vi "MSE310ProjectV2.vi"() -> ()   [LabVIEW 2016]
uses:
  MSE310Project-master/MSE310 Project Control.ctl
  <vilib>/DAQmx/read.llb/DAQmx Read (Digital Bool 1Line 1Point).vi
  <vilib>/DAQmx/write.llb/DAQmx Write (Digital Bool 1Line 1Point).vi
  <vilib>/DAQmx/create/channels.llb/DAQmx Create Channel (DO-Digital Output).vi
  <vilib>/DAQmx/create/channels.llb/DAQmx Create Channel (DI-Digital Input).vi
  <vilib>/DAQmx/miscellaneous.llb/DAQmx Fill In Error Info.vi
panel:
  out "KICK_GT1":bool
  out "HOP_DELAY":u16
  out "TIME_HOP":u16
  out "TIME_CUR":u16
  out "HOPPER-1":bool
  out "HOPPER":bool
  out "HOP_TIME_FLAG":bool
  out "KICK_E1":bool
  out "TOP_PUSH-1":bool
  out "KICK_FLAG-1":bool
  out "KICK_FLAG":bool
  out "KICK_COUNT":u16
  out "HOP_LIT_SENS":bool
  out "TOP_PUSH":bool
  out "RUNNING":bool
  out "START":bool
  out "TOP_LIT_SENS":bool
  out "TOP_MAT_SENS":bool
  out "STOP":T1
  in  "stop":bool
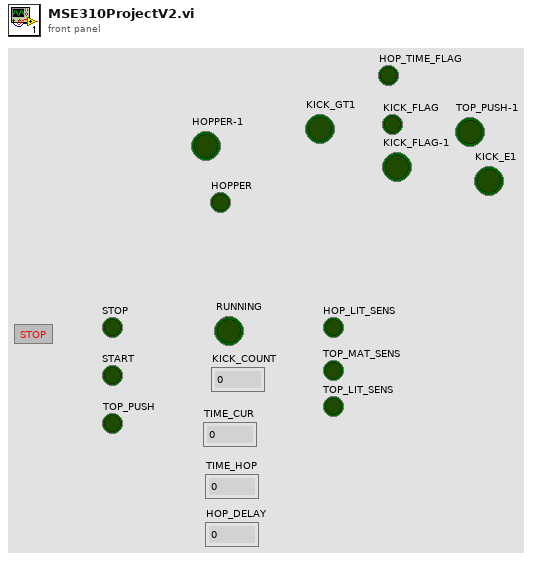
[diagram p1: front panel]
types:
  T1 = typedef "MSE310 Project Control.ctl" = bool
  T2 = cluster{"task out":refnum<k21>, "error out":errorcluster, "task out":refnum<k21>, "error out":errorcluster, "task out":refnum<k21>, "error out":errorcluster, "task out":refnum<k21>, "error out":errorcluster}
  T3 = cluster{"task out":refnum<k21>, "error out":errorcluster, "task out":refnum<k21>, "error out":errorcluster, "task out":refnum<k21>, "error out":errorcluster, "task out":refnum<k21>, "error out":errorcluster, "task out":refnum<k21>, "error out":errorcluster}
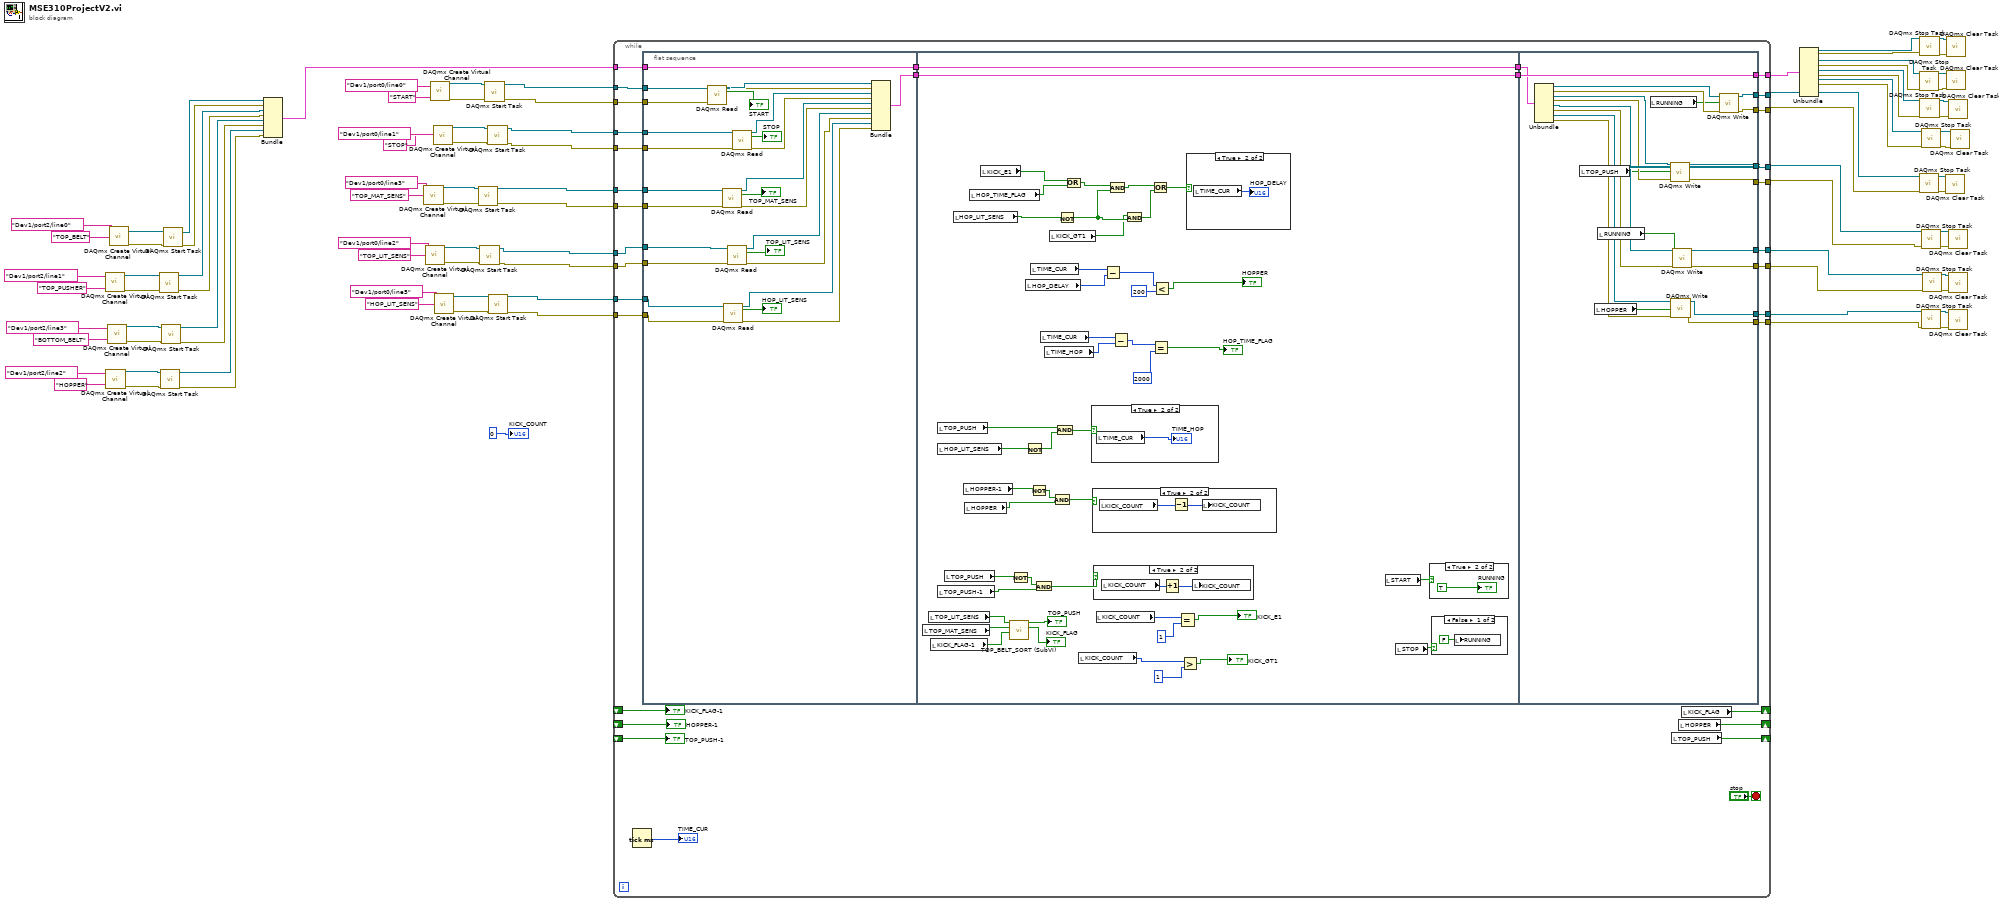
[diagram p0: block diagram]
diagram:
  n1 = call-poly <vilib>:"DAQmx Create Virtual Channel.vi"("lines"=tag "Dev1/port2/line1", "name to assign"="TOP_PUSHER") -> ("task out"=w84:refnum<k21>, "error out"=w85:errorcluster)  [unwired: 12 in]
  n2 = call-poly <vilib>:"DAQmx Create Virtual Channel.vi"("lines"=tag "Dev1/port2/line2", "name to assign"="HOPPER") -> ("task out"=w9:refnum<k21>, "error out"=w10:errorcluster)  [unwired: 12 in]
  n3 = call-poly <vilib>:"DAQmx Create Virtual Channel.vi"("lines"=tag "Dev1/port2/line3", "name to assign"="BOTTOM_BELT") -> ("task out"=w31:refnum<k21>, "error out"=w32:errorcluster)  [unwired: 12 in]
  n4 = call-poly <vilib>:"DAQmx Create Virtual Channel.vi"("lines"=tag "Dev1/port2/line0", "name to assign"="TOP_BELT") -> ("task out"=w76:refnum<k21>, "error out"=w77:errorcluster)  [unwired: 12 in]
  n5 = call <vilib>:"DAQmx Start Task.vi"("task/channels in"=w84, "error in"=w85) -> ("task out"=w44:refnum<k21>, "error out"=w43:errorcluster)  [unwired: 12 in]
  n6 = call <vilib>:"DAQmx Start Task.vi"("task/channels in"=w9, "error in"=w10) -> ("task out"=w7:refnum<k21>, "error out"=w6:errorcluster)  [unwired: 12 in]
  n7 = call <vilib>:"DAQmx Start Task.vi"("task/channels in"=w31, "error in"=w32) -> ("task out"=w30:refnum<k21>, "error out"=w29:errorcluster)  [unwired: 12 in]
  n8 = call <vilib>:"DAQmx Start Task.vi"("task/channels in"=w76, "error in"=w77) -> ("task out"=w46:refnum<k21>, "error out"=w45:errorcluster)  [unwired: 12 in]
  n9 = Bundle("task out"=w46, "error out"=w45, "task out"=w44, "error out"=w43, "task out"=w30, "error out"=w29, "task out"=w7, "error out"=w6) -> (w42:T2)  [unwired: 1 in]
  n10 = call-poly <vilib>:"DAQmx Create Virtual Channel.vi"("lines"=tag "Dev1/port0/line3", "name to assign"="TOP_MAT_SENS") -> ("task out"=w81:refnum<k21>, "error out"=w82:errorcluster)  [unwired: 12 in]
  n11 = call-poly <vilib>:"DAQmx Create Virtual Channel.vi"("lines"=tag "Dev1/port0/line2", "name to assign"="TOP_LIT_SENS") -> ("task out"=w87:refnum<k21>, "error out"=w88:errorcluster)  [unwired: 12 in]
  n12 = call-poly <vilib>:"DAQmx Create Virtual Channel.vi"("lines"=tag "Dev1/port0/line0", "name to assign"="START") -> ("task out"=w72:refnum<k21>, "error out"=w73:errorcluster)  [unwired: 12 in]
  n13 = call-poly <vilib>:"DAQmx Create Virtual Channel.vi"("lines"=tag "Dev1/port0/line1", "name to assign"="STOP") -> ("task out"=w74:refnum<k21>, "error out"=w75:errorcluster)  [unwired: 12 in]
  n14 = call-poly <vilib>:"DAQmx Create Virtual Channel.vi"("lines"=tag "Dev1/port0/line5", "name to assign"="HOP_LIT_SENS") -> ("task out"=w15:refnum<k21>, "error out"=w16:errorcluster)  [unwired: 12 in]
  n15 = call <vilib>:"DAQmx Start Task.vi"("task/channels in"=w81, "error in"=w82) -> ("task out"=w69:refnum<k21>, "error out"=w68:errorcluster)  [unwired: 12 in]
  n16 = call <vilib>:"DAQmx Start Task.vi"("task/channels in"=w87, "error in"=w88) -> ("task out"=w67:refnum<k21>, "error out"=w66:errorcluster)  [unwired: 12 in]
  n17 = call <vilib>:"DAQmx Start Task.vi"("task/channels in"=w72, "error in"=w73) -> ("task out"=w65:refnum<k21>, "error out"=w64:errorcluster)  [unwired: 12 in]
  n18 = call <vilib>:"DAQmx Start Task.vi"("task/channels in"=w74, "error in"=w75) -> ("task out"=w71:refnum<k21>, "error out"=w70:errorcluster)  [unwired: 12 in]
  n19 = call <vilib>:"DAQmx Start Task.vi"("task/channels in"=w15, "error in"=w16) -> ("task out"=w13:refnum<k21>, "error out"=w12:errorcluster)  [unwired: 12 in]
  n20 = while {
    tunnel: w71 -> [w120]
    tunnel: w70 -> [w119]
    tunnel: w69 -> [w118]
    tunnel: w68 -> [w117]
    tunnel: w67 -> [w116]
    tunnel: w66 -> [w115]
    tunnel: w65 -> [w114]
    tunnel: w64 -> [w113]
    tunnel: [w112] -> w63
    tunnel: w42 -> [w107]
    tunnel: [w106] -> w40
    tunnel: [w105] -> w39
    tunnel: [w104] -> w35
    tunnel: [w103] -> w34
    tunnel: [w102] -> w26
    tunnel: [w101] -> w25
    shift-right: [w96] -> _
    shift-left: _ -> [w95]
    tunnel: w13 -> [w100]
    tunnel: w12 -> [w99]
    tunnel: [w98] -> w3
    tunnel: [w97] -> w2
    shift-right: [w94] -> _
    shift-left: _ -> [w91]
    shift-right: [w93] -> _
    shift-left: _ -> [w92]
    stop <- "stop" stop-if-true
    n21 = Tick Count (ms)() -> (millisecond timer value=→"TIME_CUR":u32)
    n22 = flat-sequence {
      tunnel: w120 -> [w148]
      tunnel: w119 -> [w147]
      tunnel: w118 -> [w145]
      tunnel: w117 -> [w144]
      tunnel: w116 -> [w143]
      tunnel: w115 -> [w142]
      tunnel: w114 -> [w139]
      tunnel: w113 -> [w138]
      tunnel: [w128] -> w110
      tunnel: [w127] -> w108
      tunnel: w107 -> [w127]
      tunnel: w100 -> [w125]
      tunnel: w99 -> [w124]
      tunnel: [w194] -> w111
      tunnel: w110 -> [w194]
      tunnel: [w193] -> w109
      tunnel: w108 -> [w193]
      tunnel: [w224] -> w112
      tunnel: w111 -> [w224]
      tunnel: w109 -> [w223]
      tunnel: [w218] -> w106
      tunnel: [w217] -> w105
      tunnel: [w216] -> w104
      tunnel: [w215] -> w103
      tunnel: [w212] -> w102
      tunnel: [w211] -> w101
      tunnel: [w205] -> w98
      tunnel: [w204] -> w97
      frame #0 {
        n23 = call-poly <vilib>:"DAQmx Read.vi"("task/channels in"=w139, "error in"=w138) -> ("task out"=w136:refnum<k21>, "data"=→"START":bool, "error out"=w135:errorcluster)  [unwired: 11 in]
        n24 = call-poly <vilib>:"DAQmx Read.vi"("task/channels in"=w145, "error in"=w144) -> ("task out"=w132:refnum<k21>, "data"=→"TOP_MAT_SENS":bool, "error out"=w131:errorcluster)  [unwired: 11 in]
        n25 = call-poly <vilib>:"DAQmx Read.vi"("task/channels in"=w125, "error in"=w124) -> ("task out"=w123:refnum<k21>, "data"=→"HOP_LIT_SENS":bool, "error out"=w122:errorcluster)  [unwired: 11 in]
        n26 = call-poly <vilib>:"DAQmx Read.vi"("task/channels in"=w143, "error in"=w142) -> ("task out"=w130:refnum<k21>, "data"=→"TOP_LIT_SENS":bool, "error out"=w129:errorcluster)  [unwired: 11 in]
        n27 = call-poly <vilib>:"DAQmx Read.vi"("task/channels in"=w148, "error in"=w147) -> ("task out"=w134:refnum<k21>, "data"=→"STOP":bool, "error out"=w133:errorcluster)  [unwired: 11 in]
        n28 = Bundle("task out"=w136, "error out"=w135, "task out"=w134, "error out"=w133, "task out"=w132, "error out"=w131, "task out"=w130, "error out"=w129, "task out"=w123, "error out"=w122) -> (w128:T3)  [unwired: 1 in]
      }
      frame #1 {
        n29 = local read "TOP_MAT_SENS"() -> (w185:bool)
        n30 = local read "TOP_LIT_SENS"() -> (w187:bool)
        n31 = local read "KICK_FLAG-1"() -> (w188:bool)
        n32 = local read "TOP_PUSH"() -> (w177:bool)
        n33 = local read "HOP_LIT_SENS"() -> (w178:bool)
        n34 = local read "TOP_PUSH-1"() -> (w179:bool)
        n35 = local read "TOP_PUSH"() -> (w180:bool)
        n36 = local read "HOP_LIT_SENS"() -> (w165:bool)
        n37 = local read "HOPPER-1"() -> (w170:bool)
        n38 = local read "HOPPER"() -> (w171:bool)
        n39 = local read "HOP_TIME_FLAG"() -> (w164:bool)
        n40 = local read "KICK_E1"() -> (w166:bool)
        n41 = call "TOP_BELT_SORT (SubVI).vi"("KICK_FLAG-1"=w188, "TOP_MAT_SENS"=w185, "TOP_LIT_SENS"=w187) -> ("Boolean"=→"KICK_FLAG":bool, "Boolean 2"=→"TOP_PUSH":bool)  [unwired: 7 in]
        n42 = Not(x=w180) -> (.not. x?=w189:bool)
        n43 = Not(x=w178) -> (.not. x?=w176:bool)
        n44 = local read "HOP_DELAY"() -> (w160:u16)
        n45 = Not(x=w170) -> (.not. x?=w168:bool)
        n46 = local read "TIME_CUR"() -> (w161:u16)
        n47 = And(x=w189, y=w179) -> (x .and. y?=w190:bool)
        n48 = local read "TIME_CUR"() -> (w174:u16)
        n49 = local read "TIME_HOP"() -> (w173:u16)
        n50 = local read "KICK_GT1"() -> (w152:bool)
        n51 = And(x=w168, y=w171) -> (x .and. y?=w169:bool)
        n52 = And(x=w177, y=w176) -> (x .and. y?=w175:bool)
        n53 = Not(x=w165) -> (.not. x?=w153:bool)
        n54 = Or(x=w166, y=w164) -> (x .or. y?=w167:bool)
        n55 = local read "KICK_COUNT"() -> (w156:u16)
        n56 = case shown="True" w175 {
          frame False {
          }
          frame True {
            n57 = local read "TIME_CUR"() -> (→"TIME_HOP":u16)
          }
        }
        n58 = case shown="True" w169 {
          frame False {
          }
          frame True {
            n59 = local read "KICK_COUNT"() -> (w197:u16)
            n60 = Decrement(x=w197) -> (x-1=w196:u16)
            n61 = local write "KICK_COUNT"(w196) -> ()
          }
        }
        n62 = case shown="True" w190 {
          frame False {
          }
          frame True {
            n63 = local read "KICK_COUNT"() -> (w200:u16)
            n64 = Increment(x=w200) -> (x+1=w199:u16)
            n65 = local write "KICK_COUNT"(w199) -> ()
          }
        }
        n66 = local read "KICK_COUNT"() -> (w182:u16)
        n67 = Subtract(x=w161, y=w160) -> (x-y=w159:u16)
        n68 = And(x=w167, y=w153) -> (x .and. y?=w150:bool)
        n69 = Subtract(x=w174, y=w173) -> (x-y=w162:u16)
        n70 = And(x=w152, y=w153) -> (x .and. y?=w151:bool)
        n71 = Or(x=w150, y=w151) -> (x .or. y?=w149:bool)
        n72 = Equal?(x=w162, y=u16 2000) -> (x = y?=→"HOP_TIME_FLAG":bool)
        n73 = Less?(x=w159, y=u16 200) -> (x < y?=→"HOPPER":bool)
        n74 = Equal?(x=w182, y=u16 1) -> (x = y?=→"KICK_E1":bool)
        n75 = Greater?(x=w156, y=u16 1) -> (0:→"KICK_GT1":bool)
        n76 = case shown="True" w149 {
          frame False {
          }
          frame True {
            n77 = local read "TIME_CUR"() -> (→"HOP_DELAY":u16)
          }
        }
        n78 = local read "START"() -> (w191:bool)
        n79 = local read "STOP"() -> (w192:T1)
        n80 = case shown="True" w191 {
          frame False {
          }
          frame True {
            "RUNNING" <- TRUE ("RUNNING")
          }
        }
        n81 = case shown="False" w192 {
          frame False {
            n82 = local write "RUNNING"(FALSE ("RUNNING")) -> ()
          }
          frame True {
          }
        }
      }
      frame #2 {
        n83 = Unbundle(w223) -> ("task out"=w222:refnum<k21>, "error out"=w221:errorcluster, "task out"=w220:refnum<k21>, "error out"=w219:errorcluster, "task out"=w214:refnum<k21>, "error out"=w213:errorcluster, "task out"=w207:refnum<k21>, "error out"=w206:errorcluster)
        n84 = local read "TOP_PUSH"() -> (w208:bool)
        n85 = local read "HOPPER"() -> (w203:bool)
        n86 = local read "RUNNING"() -> (w209:bool)
        n87 = local read "RUNNING"() -> (w210:bool)
        n88 = call-poly <vilib>:"DAQmx Write.vi"("task/channels in"=w220, "data"=w208, "error in"=w219) -> ("task out"=w216:refnum<k21>, "error out"=w215:errorcluster)  [unwired: 10 in, 1 out]
        n89 = call-poly <vilib>:"DAQmx Write.vi"("task/channels in"=w207, "data"=w203, "error in"=w206) -> ("task out"=w205:refnum<k21>, "error out"=w204:errorcluster)  [unwired: 10 in, 1 out]
        n90 = call-poly <vilib>:"DAQmx Write.vi"("task/channels in"=w214, "data"=w209, "error in"=w213) -> ("task out"=w212:refnum<k21>, "error out"=w211:errorcluster)  [unwired: 10 in, 1 out]
        n91 = call-poly <vilib>:"DAQmx Write.vi"("task/channels in"=w222, "data"=w210, "error in"=w221) -> ("task out"=w218:refnum<k21>, "error out"=w217:errorcluster)  [unwired: 10 in, 1 out]
      }
    }
    n92 = local read "TOP_PUSH"() -> (w93:bool)
    n93 = local read "HOPPER"() -> (w94:bool)
    n94 = local read "KICK_FLAG"() -> (w96:bool)
    "KICK_FLAG-1" <- w95
    "TOP_PUSH-1" <- w92
    "HOPPER-1" <- w91
  }
  n95 = Unbundle(w63) -> ("task out"=w60:refnum<k21>, "error out"=w59:errorcluster, "task out"=w56:refnum<k21>, "error out"=w55:errorcluster, "task out"=w50:refnum<k21>, "error out"=w49:errorcluster, "task out"=w48:refnum<k21>, "error out"=w47:errorcluster)  [unwired: 2 out]
  n96 = call <vilib>:"DAQmx Stop Task.vi"("task/channels in"=w56, "error in"=w55) -> ("task out"=w58:refnum<k21>, "error out"=w57:errorcluster)  [unwired: 12 in]
  n97 = call <vilib>:"DAQmx Stop Task.vi"("task/channels in"=w40, "error in"=w39) -> ("task out"=w41:refnum<k21>, "error out"=w37:errorcluster)  [unwired: 12 in]
  n98 = call <vilib>:"DAQmx Stop Task.vi"("task/channels in"=w60, "error in"=w59) -> ("task out"=w62:refnum<k21>, "error out"=w61:errorcluster)  [unwired: 12 in]
  n99 = call <vilib>:"DAQmx Stop Task.vi"("task/channels in"=w50, "error in"=w49) -> ("task out"=w54:refnum<k21>, "error out"=w53:errorcluster)  [unwired: 12 in]
  n100 = call <vilib>:"DAQmx Stop Task.vi"("task/channels in"=w48, "error in"=w47) -> ("task out"=w52:refnum<k21>, "error out"=w51:errorcluster)  [unwired: 12 in]
  n101 = call <vilib>:"DAQmx Stop Task.vi"("task/channels in"=w35, "error in"=w34) -> ("task out"=w38:refnum<k21>, "error out"=w36:errorcluster)  [unwired: 12 in]
  n102 = call <vilib>:"DAQmx Stop Task.vi"("task/channels in"=w3, "error in"=w2) -> ("task out"=w5:refnum<k21>, "error out"=w4:errorcluster)  [unwired: 12 in]
  n103 = call <vilib>:"DAQmx Stop Task.vi"("task/channels in"=w26, "error in"=w25) -> ("task out"=w28:refnum<k21>, "error out"=w27:errorcluster)  [unwired: 12 in]
  n104 = call <vilib>:"DAQmx Clear Task.vi"("task in"=w41, "error in"=w37) -> ()  [unwired: 13 in, 1 out]
  n105 = call <vilib>:"DAQmx Clear Task.vi"("task in"=w62, "error in"=w61) -> ()  [unwired: 13 in, 1 out]
  n106 = call <vilib>:"DAQmx Clear Task.vi"("task in"=w58, "error in"=w57) -> ()  [unwired: 13 in, 1 out]
  n107 = call <vilib>:"DAQmx Clear Task.vi"("task in"=w54, "error in"=w53) -> ()  [unwired: 13 in, 1 out]
  n108 = call <vilib>:"DAQmx Clear Task.vi"("task in"=w38, "error in"=w36) -> ()  [unwired: 13 in, 1 out]
  n109 = call <vilib>:"DAQmx Clear Task.vi"("task in"=w5, "error in"=w4) -> ()  [unwired: 13 in, 1 out]
  n110 = call <vilib>:"DAQmx Clear Task.vi"("task in"=w28, "error in"=w27) -> ()  [unwired: 13 in, 1 out]
  n111 = call <vilib>:"DAQmx Clear Task.vi"("task in"=w52, "error in"=w51) -> ()  [unwired: 13 in, 1 out]
  "KICK_COUNT" <- u16 0 ("KICK_COUNT")
